vi "SetLoopCounts.vi"() -> (3 "LoopCountsOut":i32)   [LabVIEW 2009]
panel:
  in  "LoopCounts":i32
  in  "Save":bool
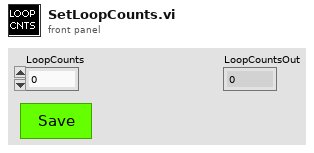
[diagram p1: front panel]
types:
  T1 = enum32{"invalid app kind", "Development System", "Run Time System", "Student Edition", "Embedded LabVIEW", "Evaluation", "Custom"}
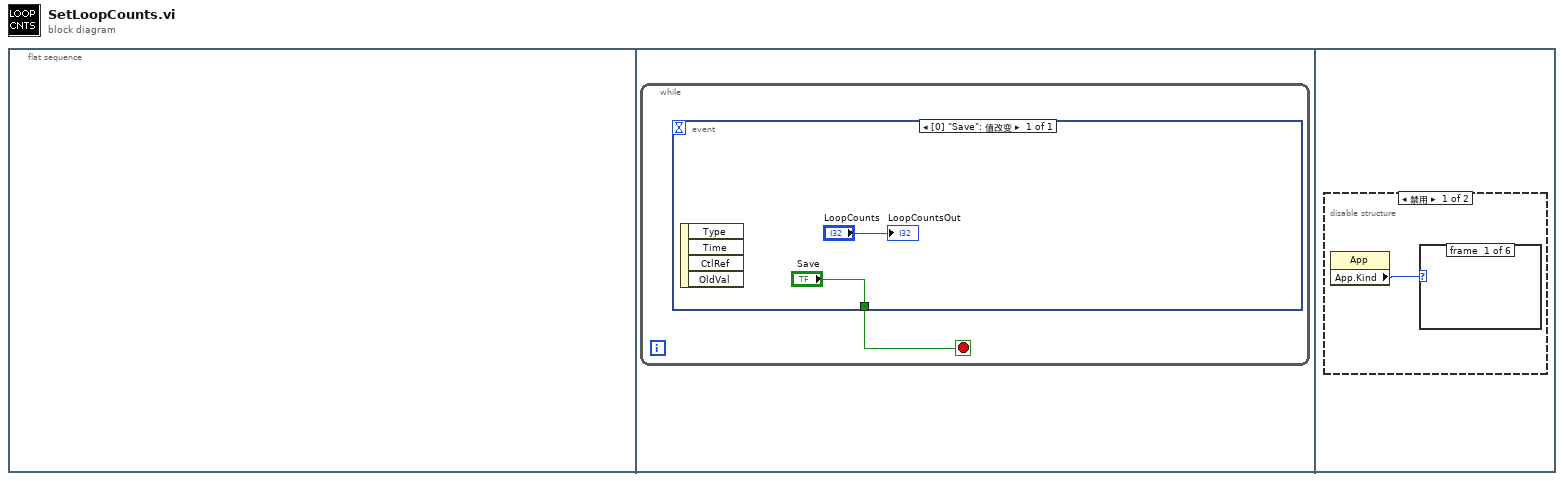
[diagram p0: block diagram]
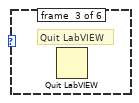
[diagram p3: hidden frame]
diagram:
  n1 = flat-sequence {
    frame #0 {
    }
    frame #1 {
      n2 = while {
        stop <- w1 stop-if-true
        n3 = event shown="[0] \"Save\": 值改变" {
          selector: _ -> [_]
          dyn-events: _ -> [_]
          timeout: _ -> [_]
          tunnel: ["Save"] -> w1
          event [0] "Save": 值改变 {
            n4 = event-data() -> ()  [unwired: 5 out]
            "LoopCountsOut" <- "LoopCounts"
          }
        }
      }
    }
    frame #2 {
      n5 = disable-structure shown="禁用" {
        frame #0 {
          n6 = property class="App"() -> ("App.Kind"=w4:T1)  [unwired: 2 in, 2 out]
          n7 = case shown="\"Run Time System\"" w4 {
            frame #0 {
            }
            frame #1 {
            }
            frame #2 {
              # "Quit LabVIEW"
              n8 = Quit LabVIEW() -> ()  [unwired: 1 in]
            }
            frame #3 {
            }
            frame #4 {
            }
            frame #5 {
            }
          }
        }
        frame #1 {
        }
      }
    }
  }
